vi "Read.vi"(7 "Read Type":T1, 8 "error in (no error)":errorcluster, 11 "NetworkStreamReader in":refnum<class "NetworkStreamReader.lvclass">) -> (0 "error out":errorcluster, 1 "New element?":bool, 2 "element":variant, 3 "NetworkStreamReader out":refnum<class "NetworkStreamReader.lvclass">)   [LabVIEW 2011, in "NetworkStreamReader.lvclass"]
doc: "Returns the requested value (either the next element available in the buffer or the most recent element). If there are no elements available in the queue, this VI will return the last valid value it returned."
uses:
  NetworkStreamReader.lvclass
  readType.ctl
  NetworkStreamReader.lvclass/NetworkStreamReader.ctl
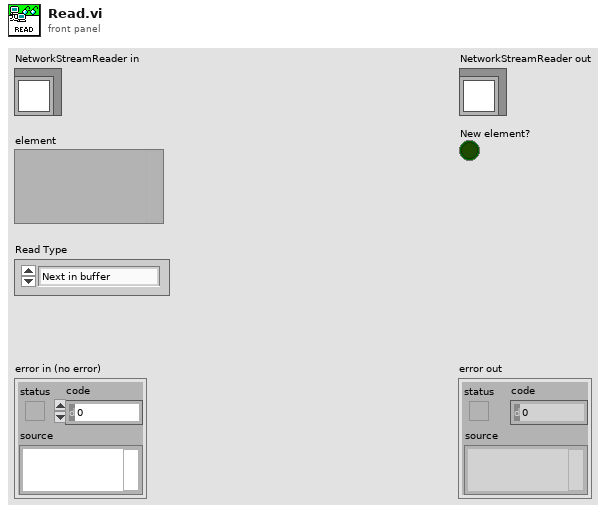
[diagram p1: front panel]
types:
  T1 = typedef "NetworkStreamReader.lvclass/readType.ctl" = enum16{"Next in buffer", "Most current"}
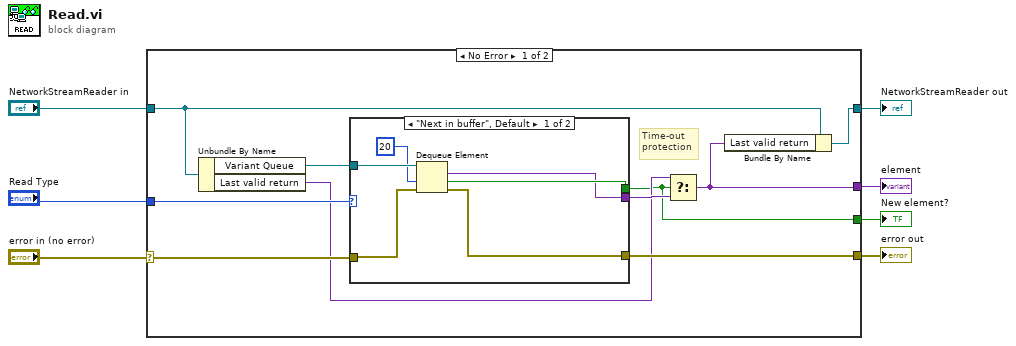
[diagram p0: block diagram]
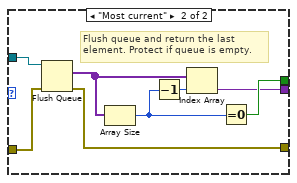
[diagram p2: hidden frame]
diagram:
  n1 = case shown="No Error" "error in (no error)" {
    selector: "error in (no error)" -> [w15 w33]
    tunnel: [w16 w33] -> w6
    tunnel: [w9 w32] -> w5
    tunnel: "NetworkStreamReader in" -> [w11 w32]
    tunnel: [w10 _] -> w4
    tunnel: "Read Type" -> [w14 _]
    tunnel: [w8 _] -> w1
    frame No Error {
      # "Time-out \nprotection"
      n2 = Unbundle By Name(w11) -> ("Variant Queue"=w17:refnum<queue>, "Last valid return"=w12:variant)
      n3 = case shown="\"Next in buffer\", Default" w14 {
        tunnel: w17 -> [w23 w31]
        tunnel: [w18 w28] -> w16
        tunnel: w15 -> [w21 w30]
        tunnel: [w20 w29] -> w8
        tunnel: [w19 w24] -> w13
        frame "Next in buffer", Default {
          n4 = Dequeue Element(queue=w23, timeout in ms (-1)=20, error in (no error)=w21) -> (element=w19:variant, timed out?=w20:bool, error out=w18:errorcluster)  [unwired: 1 out]
        }
        frame "Most current" {
          # "Flush queue and return the last\nelement. Protect if queue is empty."
          n5 = Flush Queue(queue=w31, error in (no error)=w30) -> (remaining elements=w26:variant[], error out=w28:errorcluster)  [unwired: 1 out]
          n6 = Array Size(array=w26) -> (size(s)=w27:i32)
          n7 = Decrement(x=w27) -> (x-1=w25:i32)
          n8 = Index Array(array=w26, index=w25) -> (element=w24:variant)
          n9 = Equal To 0?(x=w27) -> (x = 0?=w29:bool)
        }
      }
      n10 = Select(t=w12, s=w8, f=w13) -> (s? t:f=w10:variant)
      n11 = Bundle By Name(cluster=w11, "Last valid return"=w10) -> (w9:refnum<class "NetworkStreamReader.lvclass">)
    }
    frame Error {
    }
  }
  "error out" <- w6
  "NetworkStreamReader out" <- w5
  "element" <- w4
  "New element?" <- w1
